vi "H5Aread_Initialize.vi"() -> (1 "State Out":T1)   [LabVIEW 2017, in "H5Aread.xnode"]
uses:
  <vilib>/UPVI/lvhdf5/attribute.llb/H5Aread.xnode
  <vilib>/UPVI/lvhdf5/attribute.llb/H5Aread/H5Aread_State.ctl
  <vilib>/UPVI/lvhdf5/xnodehelpers/TermsPlus.ctl
  <vilib>/XNodeSupport/XNodeTerm3.ctl
  <vilib>/XNodeSupport/XNodeString.ctl
  <vilib>/XNodeSupport/XNodeVariant.ctl
  <vilib>/XNodeSupport/XNodeRect32.ctl
  <vilib>/XNodeSupport/XNodeInt.ctl
  <vilib>/XNodeSupport/XNodeBool.ctl
  <vilib>/XNodeSupport/XNodeTermDirection.ctl
  <vilib>/UPVI/lvhdf5/xnodehelpers/TermBehavior.ctl
  <vilib>/XNodeSupport/XNodeError3Array.ctl
  <vilib>/XNodeSupport/XNodeError3.ctl
  <vilib>/XNodeSupport/NI_XNodeSupport.lvlib
panel:
  # "LVHDF5 Toolkit\nCopyright (c) 2005-2013 by Jason D. Sommerville\nCopyright (c) 2014 by UPVI, LLC.\n\nThis use and distribution of this file is governed by the terms found in \nLICENSE.txt distributed with this toolkit and installed at\n <user.lib>\\_lvhdf5\\LICENSE.txt"
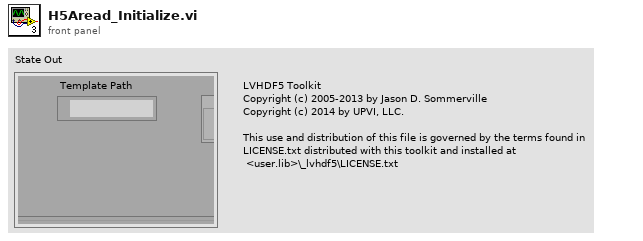
[diagram p1: front panel]
types:
  T1 = typedef "H5Aread.xnode/H5Aread_State.ctl" = cluster{"Template Path":path, "Template Ref":refnum<vi>, "Terms":T2[], "Display Name":string, "Image":picture, "Errors":T11, "Generated?":bool}
  T2 = typedef "TermsPlus.ctl" = cluster{"Term 3":T3, "Default Type":variant, "Behavior":T10, "Behavior Arg":string, "WiredResponse":bool, "Wired":enum16{"Unknown", "Unwired", "Wired"}}
  T3 = typedef "NI_XNodeSupport.lvlib/XNodeTerm3.ctl" = cluster{"Name":T4, "Id":T4, "Type":T5, "Bounds":T6, "Input?":T8, "Required?":T8, "Recommended?":T8, "Adaptive?":T8, "Hidden?":T8, "Direction":T9, "Break Wire?":T8}
  T4 = typedef "NI_XNodeSupport.lvlib/XNodeString.ctl" = string
  T5 = typedef "NI_XNodeSupport.lvlib/XNodeVariant.ctl" = variant
  T6 = typedef "NI_XNodeSupport.lvlib/XNodeRect32.ctl" = cluster{"Left":T7, "Top":T7, "Right":T7, "Bottom":T7}
  T7 = typedef "NI_XNodeSupport.lvlib/XNodeInt.ctl" = i32
  T8 = typedef "NI_XNodeSupport.lvlib/XNodeBool.ctl" = bool
  T9 = typedef "NI_XNodeSupport.lvlib/XNodeTermDirection.ctl" = enum32{"Auto", "Up", "Down", "Left", "Right", "Center"}
  T10 = typedef "TermBehavior.ctl" = enum16{"Normal", "Anything", "LVType", "Path or Ref", "Attr Name", "Attr Poly", "Elt Poly", "Dset Poly", "WDT Poly"}
  T11 = typedef "NI_XNodeSupport.lvlib/XNodeError3Array.ctl" = T12[]
  T12 = typedef "NI_XNodeSupport.lvlib/XNodeError3.ctl" = cluster{"Error":T4, "Details":T4, "Help File":T4, "Help Topic":T4}
  T13 = typedef "imagedata.ctl" = cluster{"image type":i32, "image depth":i32, "image":u8[], "mask":u8[], "colors":u32[], "Rectangle":cluster{"left":i16, "top":i16, "right":i16, "bottom":i16}}
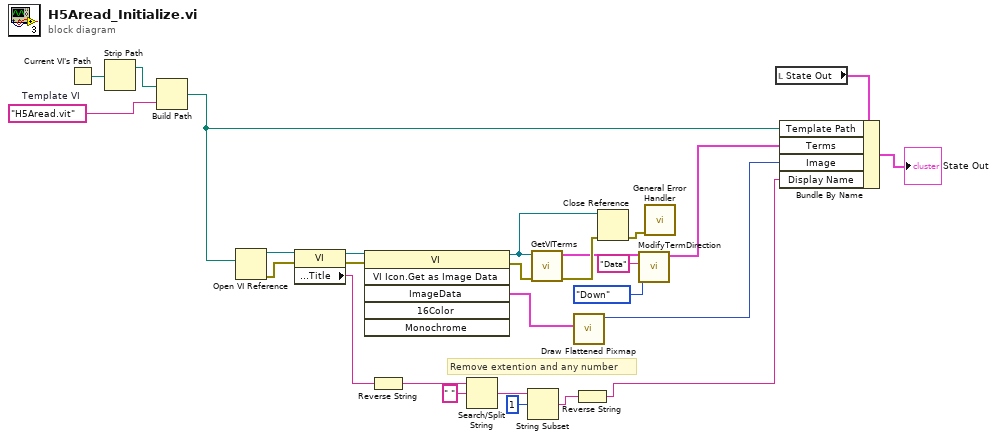
[diagram p0: block diagram]
diagram:
  w24 = "H5Aread.vit"  # Template VI
  # "Remove extention and any number"
  n1 = Current VI's Path() -> (path=w26:path)
  n2 = Strip Path(path=w26) -> (stripped path=w25:path)  [unwired: 1 out]
  n3 = Build Path(base path=w25, name or relative path=w24) -> (appended path=w22:path)
  n4 = Open VI Reference(vi path=w22) -> (vi reference=w17:refnum<vi>, error out=w18:errorcluster)  [unwired: 5 in]
  n5 = property class="VI"(reference=w17, error in=w18) -> (reference out=w15:refnum<vi>, error out=w16:errorcluster, "Front Panel.Title"=w6:string)
  n6 = invoke class="VI" method="VI Icon.Get as Image Data"(reference=w15, error in=w16) -> (reference out=w14:refnum<vi>, error out=w13:errorcluster, "ImageData"=w19:T13)  [unwired: 4 in, 3 out]
  n7 = Reverse String(1:w6) -> (0:w11:string)
  n8 = Search/Split String(string=w11, search string/char (-)=" ") -> (match + rest of string=w9:string)  [unwired: 1 in, 2 out]
  n9 = String Subset(string=w9, offset (0)=1) -> (substring=w7:string)  [unwired: 1 in]
  n10 = call <vilib>:"GetVITerms.vi"("error in (no error)"=w13, "Template Ref"=w14) -> ("error out"=w21:errorcluster, "Terms"=w4:T2[])  [unwired: 8 in]
  n11 = call <vilib>:"Draw Flattened Pixmap.vi"("image data"=w19) -> ("new picture"=w12:picture)  [unwired: 8 in]
  n12 = Reverse String(1:w7) -> (0:w5:string)
  n13 = Close Reference(reference=w14, error in (no error)=w21) -> (error out=w20:errorcluster)
  n14 = call <vilib>:"ModifyTermDirection.vi"("Term 3.Direction"=XNodeTermDirection."Down", "Id"=T4 "Data", "Terms"=w4) -> ("Terms out"=w3:T2[])  [unwired: 7 in, 1 out]
  n15 = call <vilib>:"General Error Handler.vi"("error in (no error)"=w20) -> ()  [unwired: 10 in, 5 out]
  n16 = local read "State Out"() -> (w27:T1)
  n17 = Bundle By Name(cluster=w27, "Template Path"=w22, "Terms"=w3, "Image"=w12, "Display Name"=w5) -> (→"State Out":T1)
